vi "get momentum-scaled.vi"(9 "Array 2":string[](array[string]), 10 "Array":refnum<vi>[](array[refnum]), 11 "MulticolumnListbox in":refnum<vi>) -> (0 "error out":errorcluster, 2 "Array 3":ext[](array[numeric]), 3 "Array 4":refnum<vi>[](array[refnum]))   [LabVIEW 2016, in "scale sub-VIs.lvlib"]
uses:
  sub-VIs/scale sub-VIs.lvlib
  <vilib>/Utility/miscctls.llb/LVRowAndColumnTypeDef.ctl
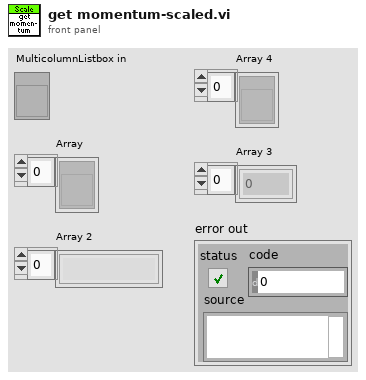
[diagram p1: front panel]
types:
  T1 = typedef "LVRowAndColumnTypeDef.ctl" = cluster{"Row":i32, "Column":i32}
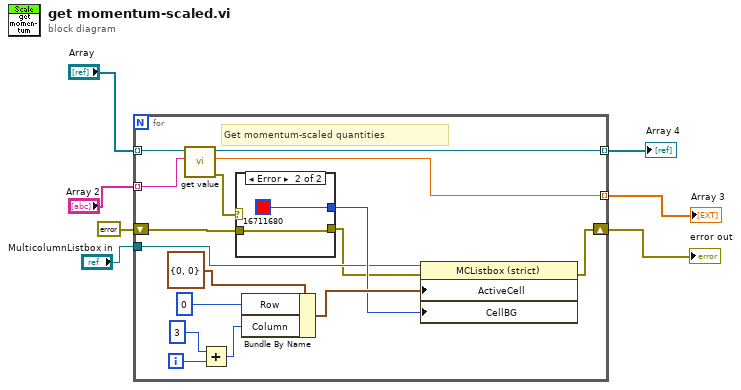
[diagram p0: block diagram]
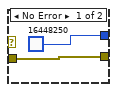
[diagram p2: hidden frame]
diagram:
  n1 = for {
    tunnel: "Array 2" -> [w11] mode=indexing
    tunnel: "Array" -> [w23] mode=indexing
    tunnel: [w22] -> w3 mode=indexing
    tunnel: [w21] -> w2 mode=indexing
    shift-right: [w9] -> w7
    shift-left: errorcluster {"status"=FALSE, "code"=0, "source"=""} ("error IO") -> [w13]
    tunnel: "MulticolumnListbox in" -> [w10]
    i -> [w19]
    # "Get momentum-scaled quantities"
    n2 = call "get value.vi"("Control Name"=w11, "VI Refnum"=w23) -> ("error out"=w15:errorcluster, "get value"=w22:ext, "VI Refnum out"=w21:refnum<vi>)  [unwired: 7 in]
    n3 = Add(x=3, y=w19) -> (x+y=w17:i32)
    n4 = case shown="Error" w15 {
      tunnel: [u32 16448250 u32 16711680] -> w14
      tunnel: [w24 w26] -> w8
      tunnel: w13 -> [w24 w26]
      frame No Error {
      }
      frame Error {
      }
    }
    n5 = Bundle By Name(cluster=T1 {"Row"=0, "Column"=0} ("Active Cell:Active Cell"), "Row"=0, "Column"=w17) -> (w20:T1)
    n6 = property on="Property Node" class="MCListbox (strict)"(reference=w10, error in=w8, "ActiveCell"=w20, "CellBG"=w14) -> (error out=w9:errorcluster)  [unwired: 1 out]
  }
  "error out" <- w7
  "Array 3" <- w3
  "Array 4" <- w2
